vi "Seperating Reference and Label.vi"(7 "Data Cluster In":T1, 8 "error in (no error)":errorcluster) -> (0 "error out":errorcluster, 5 "Data Cluster Out":T1)   [LabVIEW 2021, in "Test Panel.lvlib"]
doc: "<b>Note:</b> This VI was modified by the <b>Validate DQMH Module</b> tool to turn off automatic error handling."
uses:
  Test Panel.lvlib
  Module Data--cluster.ctl
  GUI Ctrl Data's--Cluster.ctl
  Rx-Mapping Data.ctl
  14e6ffd3-0e5d-4d4c-a9c3-bccf609c9285.vi
  e108a2ea-be35-4a89-a3a5-c9c6014299e5.vi
panel:
  out "String Labele's":string[](array[string])
  out "Digital Label's":string[](array[string])
  out "Bollean Label's":string[](array[string])
  out "Class ID Wihtout Repeating":u32[](array[numeric])
  out "Class Name Without Repeating":string[](array[string])
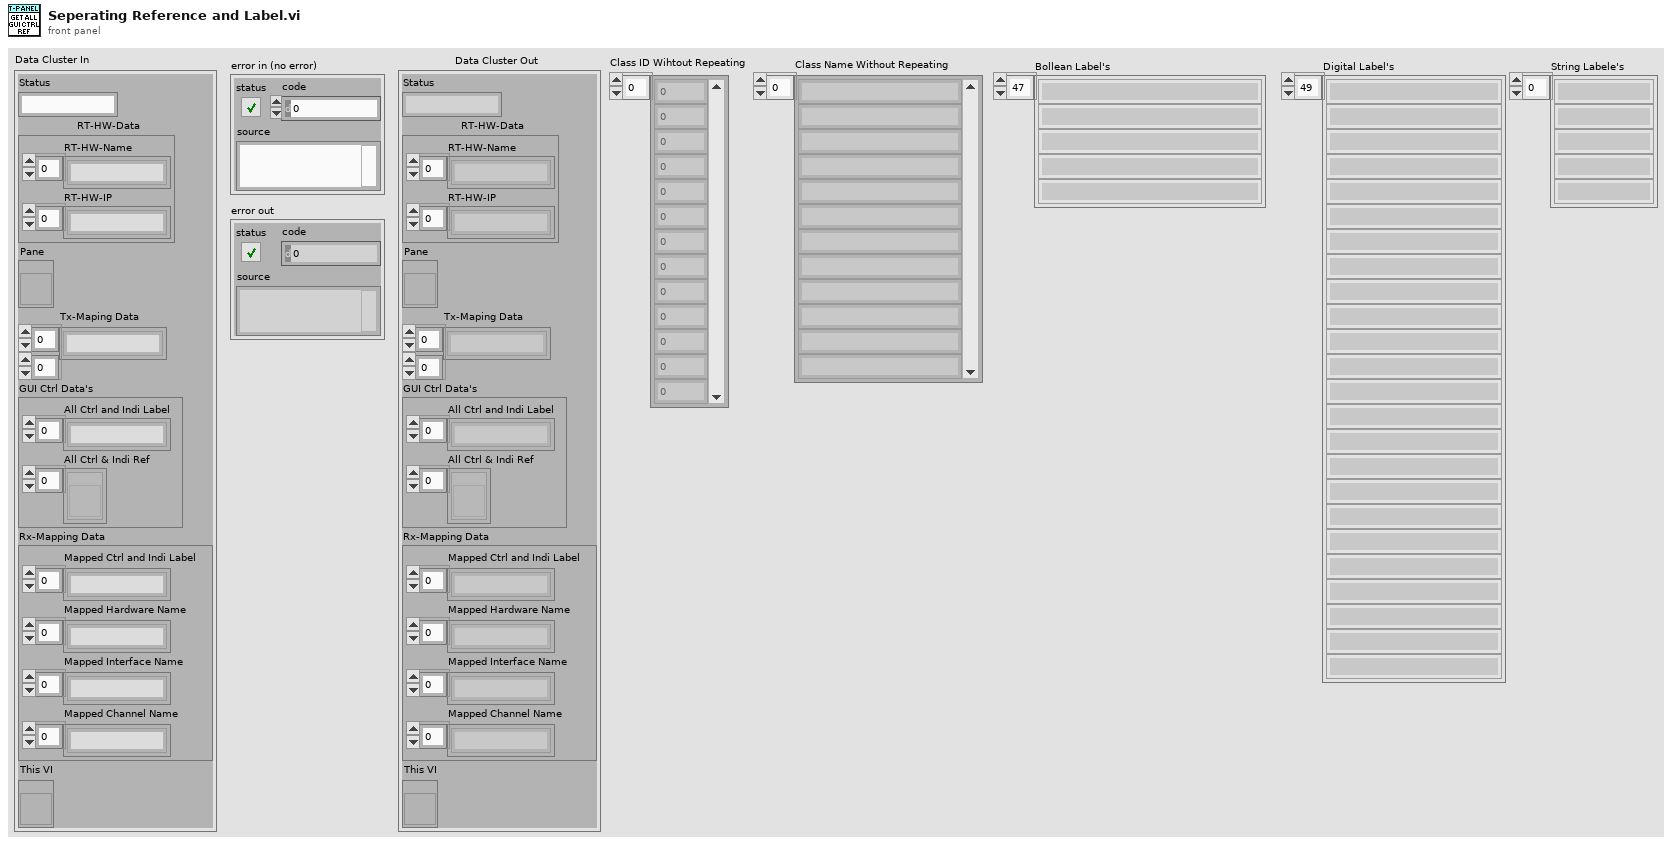
[diagram p1: front panel]
types:
  T1 = typedef "Test Panel.lvlib/Module Data--cluster.ctl" = cluster{"Status":string, "RT-HW-Data":cluster{"RT-HW-Name":string[], "RT-HW-IP":string[]}, "Pane":refnum<vi>, "Tx-Maping Data":string[][], "GUI Ctrl Data's":T2, "Rx-Mapping Data":T3, "This VI":refnum<vi>}
  T2 = typedef "Test Panel.lvlib/GUI Ctrl Data's--Cluster.ctl" = cluster{"All Ctrl and Indi Label":string[], "All Ctrl & Indi Ref":refnum<vi>[]}
  T3 = typedef "Test Panel.lvlib/Rx-Mapping Data.ctl" = cluster{"Mapped Ctrl and Indi Label":string[], "Mapped Hardware Name":string[], "Mapped Interface Name":string[], "Mapped Channel Name":string[]}
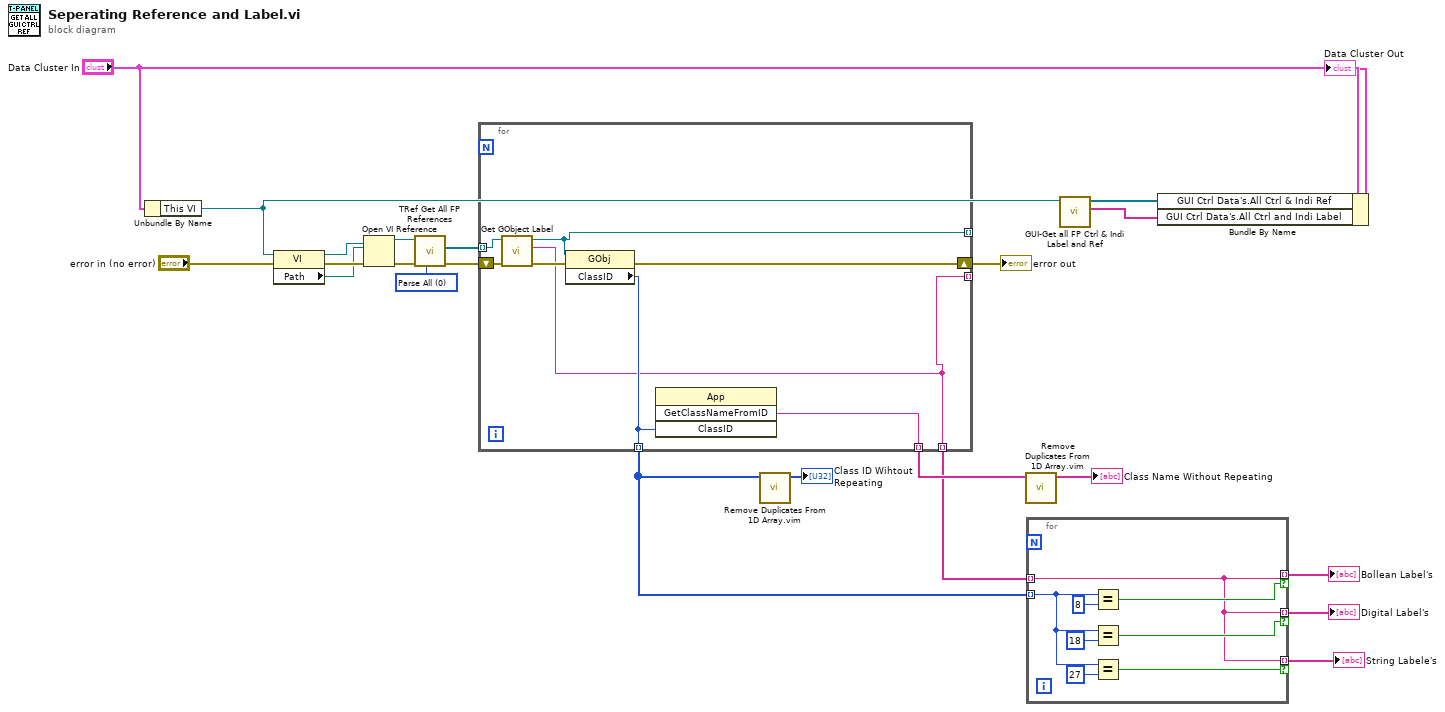
[diagram p0: block diagram]
diagram:
  w12 = u16 0 items=["Parse All", "Parse Tabs Only"] ("Parsing Rule")
  n1 = Unbundle By Name("Data Cluster In") -> ("This VI"=w3:refnum<vi>)
  n2 = property class="VI"(reference=w3, error in="error in (no error)") -> (reference out=w10:refnum<vi>, error out=w9:errorcluster, "Path"=w8:path)
  n3 = Open VI Reference(type specifier VI Refnum (for type only)=w10, vi path=w8, error in (no error)=w9) -> (vi reference=w7:refnum<vi>, error out=w6:errorcluster)  [unwired: 3 in]
  n4 = call <vilib>:"TRef Get All FP References.vi"("Parsing Rule"=w12, "error in (no error)"=w6, "VI Refnum"=w7) -> ("error out"=w5:errorcluster, "All FP Objects"=w4:refnum<vi>[])  [unwired: 4 in, 3 out]
  n5 = for {
    tunnel: [w26] -> _ mode=indexing
    shift-right: [w25] -> w21
    shift-left: w5 -> [w29]
    tunnel: [w26] -> w13 mode=indexing
    tunnel: [w31] -> w18 mode=indexing
    tunnel: [w30] -> w17 mode=indexing
    tunnel: w4 -> [w27] mode=indexing
    tunnel: [w24] -> _ mode=indexing
    n6 = call <vilib>:"Get GObject Label.vi"("error in (no error)"=w29, "GObject"=w27) -> ("error out"=w28:errorcluster, "Object Label"=w26:string, "dup GObject"=w24:refnum<vi>)  [unwired: 5 in, 2 out]
    n7 = property class="GObj"(reference=w24, error in=w28) -> (error out=w25:errorcluster, "ClassID"=w30:u32)  [unwired: 1 out]
    n8 = invoke class="App" method="GetClassNameFromID"("ClassID"=w30) -> ("GetClassNameFromID"=w31:string)  [unwired: 3 in, 3 out]
  }
  "error out" <- w21
  n9 = call "Remove Duplicates From 1D Array.vim"("array"=w17) -> ("array with duplicates removed"=→"Class ID Wihtout Repeating":u32[])  [unwired: 10 in]
  n10 = call "Remove Duplicates From 1D Array.vim"("array"=w18) -> ("array with duplicates removed"=→"Class Name Without Repeating":string[])  [unwired: 10 in]
  n11 = for {
    tunnel: w13 -> [w33] mode=indexing
    tunnel: w17 -> [w34] mode=indexing
    tunnel: [w33] -> w16 mode=indexing if=w37
    tunnel: [w33] -> w15 mode=indexing if=w36
    tunnel: [w33] -> w14 mode=indexing if=w32
    n12 = Equal?(x=w34, y=u32 8) -> (x = y?=w37:bool)
    n13 = Equal?(x=w34, y=u32 18) -> (x = y?=w36:bool)
    n14 = Equal?(x=w34, y=u32 27) -> (x = y?=w32:bool)
  }
  "Bollean Label's" <- w16
  "Digital Label's" <- w15
  "String Labele's" <- w14
  n15 = call "GUI-Get all FP Ctrl & Indi Label and Ref.vi"("Respected VI Ref"=w3) -> ("All Object Label"=w1:string[], "All Object Ref"=w2:refnum<vi>[])  [unwired: 9 in]
  n16 = Bundle By Name(cluster="Data Cluster In", "GUI Ctrl Data's.All Ctrl & Indi Ref"=w2, "GUI Ctrl Data's.All Ctrl and Indi Label"=w1) -> (→"Data Cluster Out":T1)
